vi "ConvertToVolts.vi"(10 "Voltage Range":dbl=10.0 format="%#_13g", 11 "Channel":i16) -> (3 "Volts":dbl)   [LabVIEW 2016]
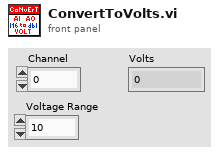
[diagram p1: front panel]
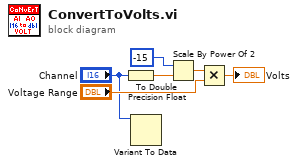
[diagram p0: block diagram]
diagram:
  n1 = To Double Precision Float(number="Channel") -> (double precision float=w2:dbl)
  n2 = Variant To Data(type="Channel", Variant="Channel") -> ()  [unwired: 1 in, 2 out]
  n3 = Scale By Power Of 2(n=i16 -15, x=w2) -> (x*2^n=w4:dbl)
  n4 = Multiply(x=w4, y="Voltage Range") -> (x*y=→"Volts":dbl)
